vi "VISA Write Async.vi"(8 "error in (no error)":errorcluster, 10 "write buffer":string, 11 "Instrument in":refnum<class "Instrument.lvclass">) -> (0 "error out":errorcluster, 2 "return count":u32, 3 "Instrument out":refnum<class "Instrument.lvclass">)   [LabVIEW 2015, in "Instrument.lvclass"]
doc: "(Dynamic) Write to this Instrument using an asynchronous VISA call. Override this method if the Instrument has communication idiosyncrasies."
uses:
  Instrument.lvclass
  Instrument.lvclass/Instrument.ctl
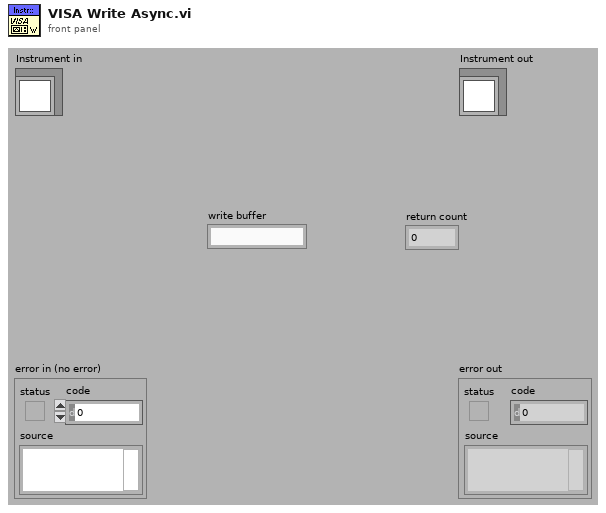
[diagram p1: front panel]
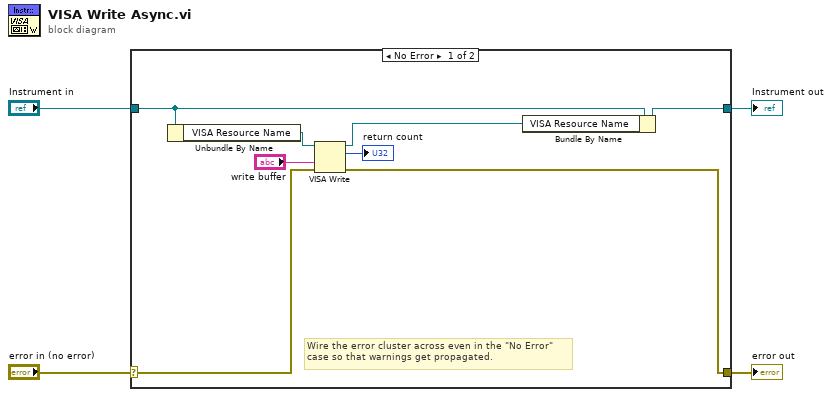
[diagram p0: block diagram]
diagram:
  n1 = case shown="No Error" "error in (no error)" {
    selector: "error in (no error)" -> [w9 w14]
    tunnel: [w8 w14] -> w3
    tunnel: [w6 w13] -> w1
    tunnel: "Instrument in" -> [w12 w13]
    frame No Error {
      # "Wire the error cluster across even in the \"No Error\"\ncase so that warnings get propagated."
      n2 = Unbundle By Name(w12) -> ("VISA Resource Name"=w11:refnum<visa-resource-name>)
      n3 = VISA Write(VISA resource name=w11, write buffer="write buffer", error in (no error)=w9) -> (VISA resource name out=w5:refnum<visa-resource-name>, return count=→"return count":u32, error out=w8:errorcluster)
      n4 = Bundle By Name(cluster=w12, "VISA Resource Name"=w5) -> (w6:refnum<class "Instrument.lvclass">)
    }
    frame Error {
    }
  }
  "error out" <- w3
  "Instrument out" <- w1
